vi "Backup Installed Source.vi"(8 "Error In":errorcluster, 9 "Backup Dir":path, 10 "LabVIEW Dir":path=path "C:/Program Files/National Instruments/LabVIEW 2013", 11 "Configuration":T1) -> (0 "Error Out":errorcluster, 2 "Archive Dest":path=path "C:/Program Files/National Instruments/LabVIEW 2013/vi.lib/LabVIEW Hacker/EZ430-Chronos-Interface-bak.zip", 3 "Configuration":T1)   [LabVIEW 2011, in "LVH-Toolbox.lvlib" / "LVH-Build-Tools.lvlib"]
doc: "Create an archived copy of the installed source components to preseve any changes in the event of a sync failure."
uses:
  LVH-Build-Tools.lvlib
  Type Defs/Configuration.ctl
  System Tools/LVH-SystemTools.lvlib
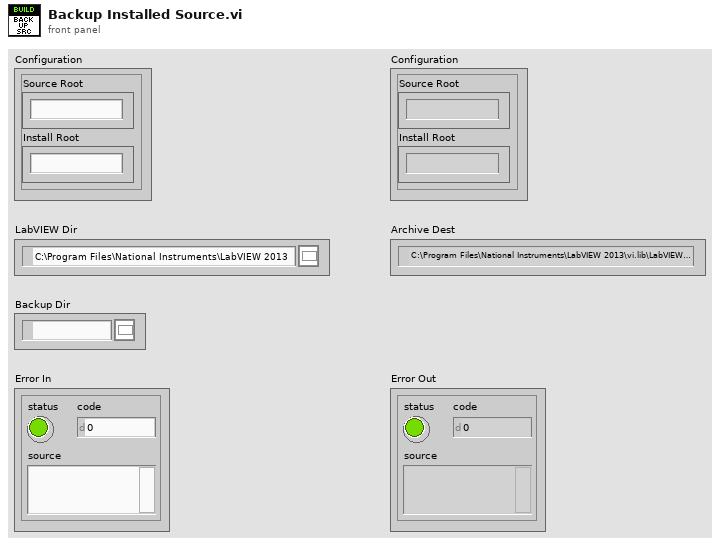
[diagram p1: front panel]
types:
  T1 = typedef "LVH-Toolbox.lvlib/LVH-Build-Tools.lvlib/Configuration.ctl" = cluster{"Source Root":string, "Install Root":string, "Components":string[], "Ignore":string[]}
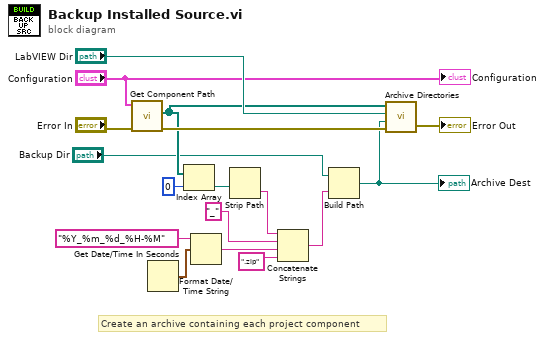
[diagram p0: block diagram]
diagram:
  # "Create an archive containing each project component"
  n1 = call "Get Component Path.vi"("Error In"="Error In", "Configuration"="Configuration") -> ("Error Out"=w16:errorcluster, "Component Install Paths"=w14:path[])  [unwired: 7 in, 1 out]
  n2 = Get Date/Time In Seconds() -> (seconds since 1Jan1904=w9:timestamp)
  n3 = Index Array(array=w14, index=0) -> (element=w12:path)
  n4 = Format Date/Time String(time format string (%c)="%Y_%m_%d_%H-%M", seconds (now)=w9) -> (date/time string=w6:string)  [unwired: 1 in]
  n5 = Strip Path(path=w12) -> (name=w4:string)  [unwired: 1 out]
  n6 = Concatenate Strings(w4, "_" ("string"), w6, ".zip" ("string")) -> (w3:string)
  n7 = Build Path(base path="Backup Dir", name or relative path=w3) -> (appended path=w2:path)
  "Archive Dest" <- w2
  n8 = call "Archive Directories.vi"("Error In"=w16, "Archive Dest"=w2, "Archive Root"="LabVIEW Dir", "Directory Paths"=w14) -> ("Error Out"=→"Error Out":errorcluster)  [unwired: 7 in]
  "Configuration" <- "Configuration"
